vi "ShutterControl.vi"(8 "error in (no error)":errorcluster, 9 "id":enum16{"1", "2", "3", "4", "all"}(ring), 10 "cmd":enum16{"off", "on"}(ring), 11 "VISA resource name":refnum<visa-resource-name>="COM11") -> (0 "error out":errorcluster)   [LabVIEW 2019]
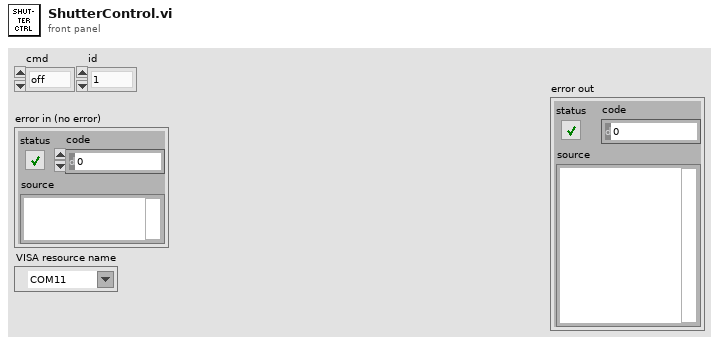
[diagram p1: front panel]
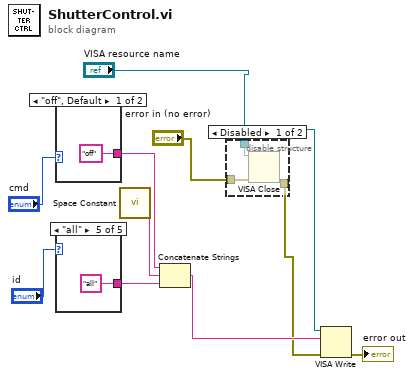
[diagram p0: block diagram]
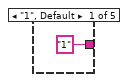
[diagram p3: hidden frame]
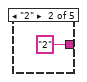
[diagram p4: hidden frame]
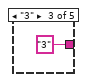
[diagram p5: hidden frame]
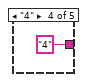
[diagram p6: hidden frame]
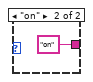
[diagram p7: hidden frame]
diagram:
  n1 = case shown="\"off\", Default" "cmd" {
    tunnel: ["off" "on" ("write buffer")] -> w7
    frame "off", Default {
    }
    frame "on" {
    }
  }
  n2 = case shown="\"all\"" "id" {
    tunnel: ["1" "2" "3" "4" "all"] -> w6
    frame "1", Default {
    }
    frame "2" {
    }
    frame "3" {
    }
    frame "4" {
    }
    frame "all" {
    }
  }
  n3 = call <vilib>:"Space Constant.vi"() -> ("String"=w5:string)
  n4 = Concatenate Strings(w7, w5, w6) -> (w4:string)
  n5 = disable-structure shown="Disabled" {
    disable-tunnel: "error in (no error)" -> [w20 _]
    disable-tunnel: [w19 _] -> w2
    disable-tunnel: "VISA resource name" -> [w18 _]
    frame Disabled {
      n6 = VISA Close(VISA resource name=w18, error in (no error)=w20) -> (error out=w19:errorcluster)
    }
    frame Enabled {
    }
  }
  n7 = VISA Write(VISA resource name="VISA resource name", write buffer=w4, error in (no error)=w2) -> (error out=→"error out":errorcluster)  [unwired: 2 out]
